vi "Save_Indicies_for_Subtrack-1.vi"(0 "[IN] Index of Origin/Problem \nPoint inside Original Track (X1)":i32, 1 "[IN] i for X1":i32, 2 "[IN] Subtrack":T1, 3 "[IN] Index of Track Conta-\nining Origin/Problem (X2)":i32, 4 "[IN] i for X2":i32) -> (5 "[OUT] Subtrack":T1)   [LabVIEW 2013]
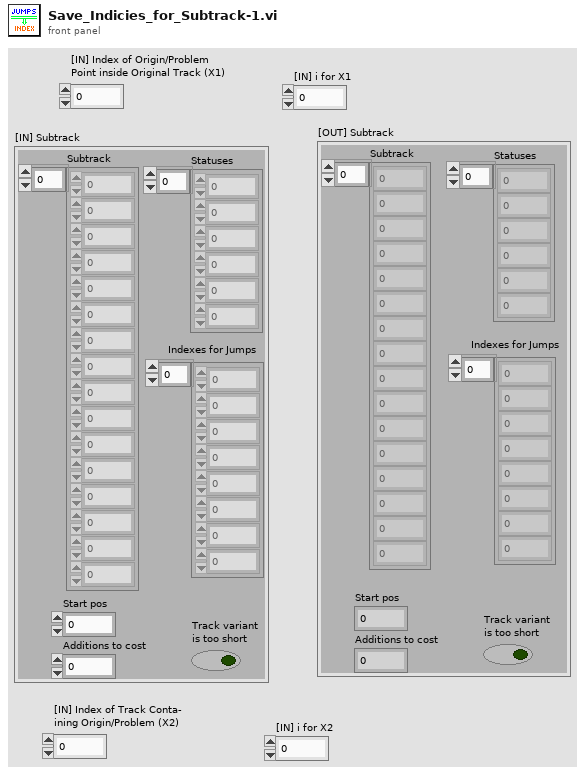
[diagram p1: front panel]
types:
  T1 = cluster{"Subtrack":dbl[], "Statuses":i16[], "Start pos":i32, "Additions to cost":i32, "Track variant \nis too short":bool, "Indexes for Jumps":i32[]}
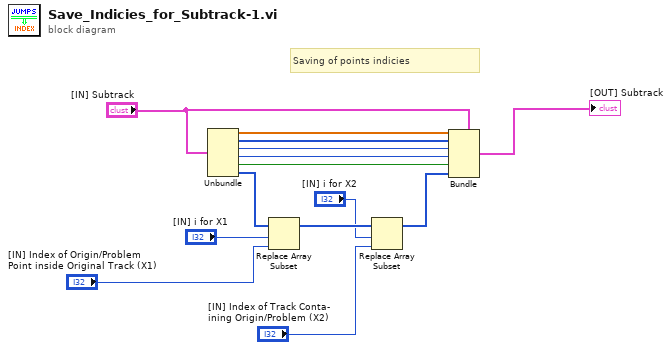
[diagram p0: block diagram]
diagram:
  # "Saving of points indicies"
  n1 = Unbundle("[IN] Subtrack") -> ("Subtrack"=w13:dbl[], "Statuses"=w12:i16[], "Start pos"=w11:i32, "Additions to cost"=w10:i32, "Track variant \nis too short"=w9:bool, "Indexes for Jumps"=w8:i32[])
  n2 = Replace Array Subset(array=w8, new element="[IN] Index of Origin/Problem \nPoint inside Original Track (X1)", index="[IN] i for X1") -> (w6:i32[])
  n3 = Replace Array Subset(array=w6, new element="[IN] Index of Track Conta-\nining Origin/Problem (X2)", index="[IN] i for X2") -> (w2:i32[])
  n4 = Bundle(cluster="[IN] Subtrack", "Subtrack"=w13, "Statuses"=w12, "Start pos"=w11, "Additions to cost"=w10, "Track variant \nis too short"=w9, "Indexes for Jumps"=w2) -> (→"[OUT] Subtrack":T1)
